vi "Pre Launch Init.vi"(11 "BuildServer in":refnum<class "BuildServer.lvclass">) -> (0 "error out":errorcluster, 3 "BuildServer out":refnum<class "BuildServer.lvclass">)   [LabVIEW 2017, in "BuildServer.lvlib" / "BuildServer.lvclass"]
doc: "(<B>Filename</B>: Actor Framework.lvlib:Actor.lvclass:Pre Launch Init.vi)\n\nDefines behavior that occurs after the Launch Nested Actor method is invoked but before the actor's Actor Core method begins running.\n\nBy default, this method does nothing. A descendant class may override it to define behavior."
uses:
  BuildServer.lvclass
  C:/Users/Public/Documents/wc/BuildFarm/src/LabVIEW/vi.lib/BenjaminR/Build Farm/Actors/Framework/Actor wLauncher/Actor wLauncher.lvclass
  C:/Program Files (x86)/National Instruments/LabVIEW 2017/vi.lib/ActorFramework/Actor/Actor.lvclass
  BuildServer.lvclass/BuildServer.ctl
  <vilib>/ActorFramework/Actor/Actor.lvclass/Actor.ctl
  <vilib>/ActorFramework/Message Enqueuer/Message Enqueuer.lvclass/Message Enqueuer.ctl
  <vilib>/ActorFramework/Message Enqueuer/Init from Existing Queue.vi
  <vilib>/ActorFramework/Message Enqueuer/Enqueue.vi
  BuildServer Messages/Launching Msg/Launching Msg.lvclass
  C:/Program Files (x86)/National Instruments/LabVIEW 2017/vi.lib/ActorFramework/Message/Message.lvclass
  <vilib>/ActorFramework/Message Priority Queue/Priority Enqueue.vi
  <vilib>/ActorFramework/Message Enqueuer/Message Enqueuer.lvclass
  Framework/Actor wHelper/Actor wHelper.lvclass
  <vilib>/BenjaminR/LookUp Table API/LUT.lvclass
  <vilib>/ActorFramework/Actor/Actor.lvclass
  Framework/Actor wLauncher/Actor wLauncher.lvclass
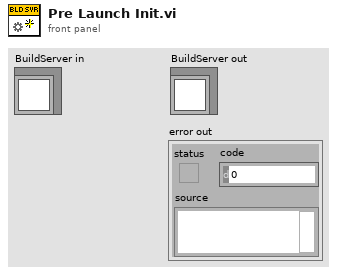
[diagram p1: front panel]
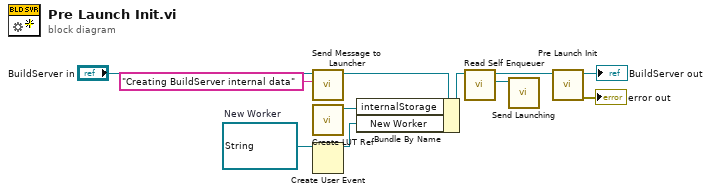
[diagram p0: block diagram]
diagram:
  w5 = refnum<user-event> refnum  # New Worker
  n1 = call "Send Message to Launcher.vi"("Msg to Launcher"="Creating BuildServer internal data", "Actor wLauncher in"="BuildServer in") -> ("Actor wLauncher out"=w2:refnum<class "BuildServer.lvclass">)  [unwired: 8 in, 1 out]
  n2 = call <vilib>:"Create LUT Ref.vi"() -> ("LUT out"=w8:refnum<class "LUT.lvclass">)  [unwired: 10 in, 1 out]
  n3 = Create User Event(user event datatype=w5) -> (user event=w4:refnum<user-event>)  [unwired: 1 in, 1 out]
  n4 = Bundle By Name(cluster=w2, "internalStorage"=w8, "New Worker"=w4) -> (w7:refnum<class "BuildServer.lvclass">)
  n5 = call <vilib>:"Read Self Enqueuer.vi"("Actor"=w7) -> ("Self Enqueuer"=w6:refnum<class "Message Enqueuer.lvclass">)  [unwired: 10 in]
  n6 = call "Send Launching.vi"("Message Enqueuer in"=w6) -> ()  [unwired: 9 in, 2 out]
  n7 = call-parent "Pre Launch Init.vi"("Actor wHelper in"=w7) -> ("error out"=→"error out":errorcluster, "Actor wHelper out"=→"BuildServer out":refnum<class "BuildServer.lvclass">)  [unwired: 9 in]
